vi "Cameras.vi"(4 "error in (no error)":errorcluster, 7 "Image Notifier":refnum<notifier>) -> ()   [LabVIEW 2015]
doc: "This VI runs in parallel to other tasks. It gets images from the camera, processes them for color or shape and use that information to affect robot behavior."
uses:
  <vilib>/Rock Robotics/WPI/Camera/WPI_CameraImageSize.ctl
  Robot Global Data.vi
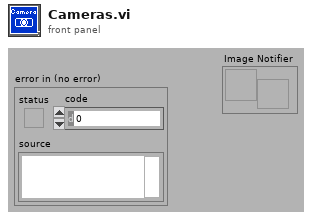
[diagram p1: front panel]
types:
  T1 = typedef "Image Type" = u32
  T2 = typedef "WPI_CameraImageSize.ctl" = enum16{"640x480", "320x240", "160x120", "Custom"}
  T3 = typedef "WPI_CameraDevRef.ctl" = cluster{"Camera Address":string, "CameraStatus":errorcluster}
  T4 = typedef "IMAQ Image.ctl" = refnum<image>
  T5 = enum16{"Update Mode", "Get Image", "Get Image Data"}
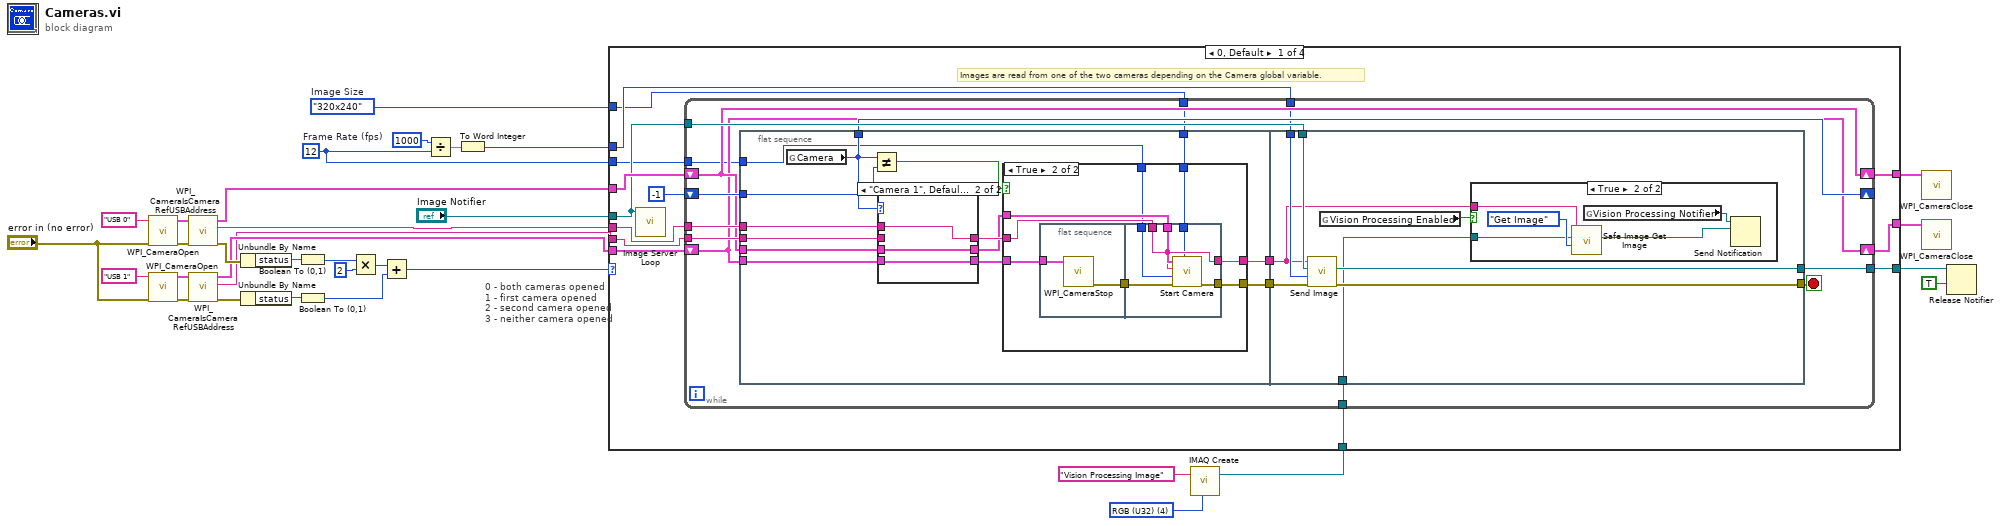
[diagram p0: block diagram]
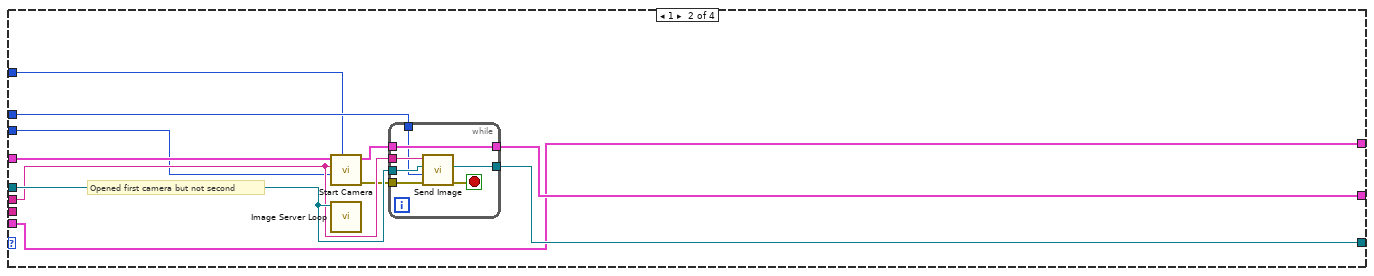
[diagram p5: hidden frame]
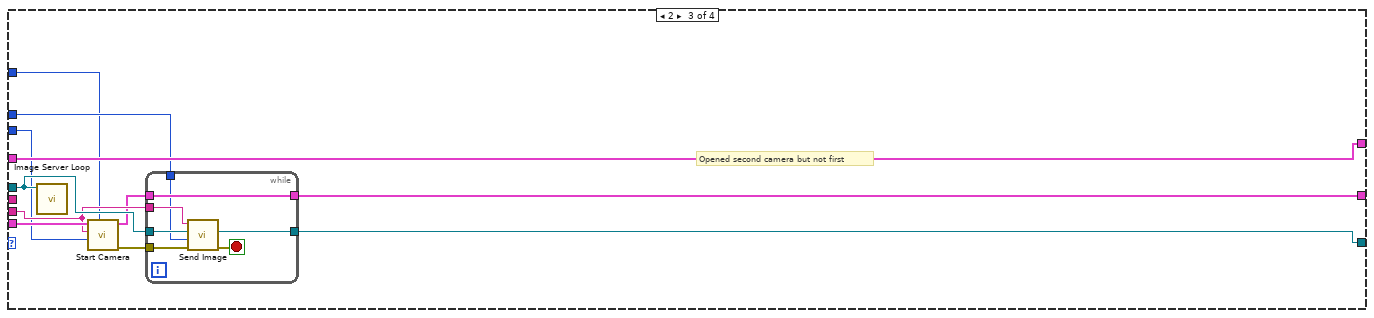
[diagram p6: hidden frame]
diagram:
  w3 = T1 4 items=["Grayscale (U8)", "Grayscale (I16)", "Grayscale (SGL)", "Complex (CSG)", "RGB (U32)", "HSL (U32)", "RGB (U64)", "Grayscale (U16)"] ("Image Type")
  w6 = 12  # Frame Rate (fps)
  w5 = WPI_CameraImageSize."320x240"  # Image Size
  n1 = call <vilib>:"WPI_CameraOpen.vi"("error in (no error)"="error in (no error)", "Camera Address"="USB 0" ("format string")) -> ("error out"=w18:errorcluster, "CameraDevRef"=w20:T3)  [unwired: 8 out]
  n2 = call <vilib>:"WPI_CameraOpen.vi"("error in (no error)"="error in (no error)", "Camera Address"="USB 1" ("format string")) -> ("error out"=w14:errorcluster, "CameraDevRef"=w16:T3)  [unwired: 8 out]
  n3 = call <vilib>:"WPI_CameraIsCameraRefUSBAddress.vi"("error in (no error)"=w18, "CameraDevRef"=w20) -> ("error out"=w17:errorcluster, "Camera Address Out"=w11:string, "CameraDevRef out"=w19:T3)  [unwired: 6 in, 1 out]
  n4 = call <vilib>:"WPI_CameraIsCameraRefUSBAddress.vi"("error in (no error)"=w14, "CameraDevRef"=w16) -> ("error out"=w13:errorcluster, "Camera Address Out"=w12:string, "CameraDevRef out"=w15:T3)  [unwired: 6 in, 1 out]
  n5 = Unbundle By Name(w17) -> ("status"=w9:bool)
  n6 = Unbundle By Name(w13) -> ("status"=w10:bool)
  n7 = Boolean To (0,1)(Boolean=w9) -> (0, 1=w24:i16)
  n8 = Boolean To (0,1)(Boolean=w10) -> (0, 1=w26:i16)
  n9 = Multiply(x=w24, y=i16 2) -> (x*y=w25:i16)
  n10 = Add(x=w25, y=w26) -> (x+y=w28:i16)
  n11 = Divide(x=1000, y=w6) -> (x/y=w7:dbl)
  n12 = To Word Integer(number=w7) -> (16bit integer=w4:i16)
  n13 = call "IMAQ Create"("Image Name"="Vision Processing Image", "Image Type"=w3) -> ("New Image"=w1:T4)  [unwired: 2 in, 2 out]
  n14 = case "0 - both cameras opened\n1 - first camera opened\n2 - second camera opened\n3 - neither camera opened" shown="0, Default" w28 {
    tunnel: [w46 w120 w137 w149] -> w33
    tunnel: "Image Notifier" -> [w39 w121 w139 w148]
    tunnel: [w45 w119 w138 w150] -> w31
    tunnel: w15 -> [w44 w119 w136 w149]
    tunnel: w19 -> [w43 w117 w138 w150]
    tunnel: w12 -> [w42 _ w135 _]
    tunnel: w11 -> [w41 w116 _ _]
    tunnel: [w40 w122 w140 w148] -> w30
    tunnel: w4 -> [w37 w114 w132 _]
    tunnel: w6 -> [w36 w113 w131 _]
    tunnel: w5 -> [w34 w112 w130 _]
    tunnel: w1 -> [w35 _ _ _]
    frame 0, Default {
      # "Images are read from one of the two cameras depending on the Camera global variable."
      n15 = call "Image Server Loop.vi"("Image Notifier"=w39) -> ()  [unwired: 11 in]
      n16 = while {
        shift-right: [w52] -> w46
        shift-left: w44 -> [w52]
        tunnel: w39 -> [w60]
        shift-right: [w53] -> w45
        shift-left: w43 -> [w53]
        tunnel: w42 -> [w56]
        tunnel: w41 -> [w57]
        tunnel: [w61] -> w40
        shift-right: [w55] -> _
        shift-left: -1 -> [w59]
        tunnel: w37 -> [w50]
        tunnel: w36 -> [w49]
        tunnel: w35 -> [w48]
        tunnel: w34 -> [w47]
        stop <- w58 stop-if-true
        n17 = flat-sequence {
          tunnel: w59 -> [w74]
          tunnel: w53 -> [w73]
          tunnel: w52 -> [w72]
          tunnel: w57 -> [w71]
          tunnel: w56 -> [w70]
          tunnel: [w64] -> w55
          tunnel: [w69] -> w54
          tunnel: [w65] -> w51
          tunnel: w49 -> [w63]
          tunnel: w47 -> [w62]
          tunnel: [w106] -> w61
          tunnel: w60 -> [w105]
          tunnel: [w104] -> w58
          tunnel: w54 -> [w103]
          tunnel: w51 -> [w101]
          tunnel: w50 -> [w102]
          tunnel: w48 -> [w100]
          frame #0 {
            n18 = global read "Robot Global Data.vi" "Camera"() -> (w64:enum16{"Camera 1", "Camera 2"})
            n19 = Not Equal?(x=w64, y=w74) -> (x != y?=w75:bool)
            n20 = case shown="\"Camera 1\", Default" w64 {
              tunnel: [w77 w81] -> w66
              tunnel: w72 -> [w78 w81]
              tunnel: [w78 w80] -> w67
              tunnel: w73 -> [w77 w80]
              tunnel: w70 -> [w76 _]
              tunnel: w71 -> [_ w79]
              tunnel: [w76 w79] -> w68
              frame "Camera 2" {
              }
              frame "Camera 1", Default {
              }
            }
            n21 = case shown="True" w75 {
              tunnel: [_ w89] -> w69
              tunnel: w68 -> [w82 w88]
              tunnel: w67 -> [_ w87]
              tunnel: w66 -> [_ w86]
              tunnel: [w82 w85] -> w65
              tunnel: w63 -> [_ w84]
              tunnel: w62 -> [_ w83]
              frame False {
              }
              frame True {
                n22 = flat-sequence {
                  tunnel: [w92] -> w90
                  tunnel: w86 -> [w91]
                  tunnel: w90 -> [w98]
                  tunnel: [w97] -> w89
                  tunnel: w88 -> [w95]
                  tunnel: w87 -> [w96]
                  tunnel: [w95] -> w85
                  tunnel: w84 -> [w94]
                  tunnel: w83 -> [w93]
                  frame #0 {
                    n23 = call <vilib>:"WPI_CameraStop.vi"("CameraDevRef"=w91) -> ("error out"=w92:errorcluster)  [unwired: 9 in, 1 out]
                  }
                  frame #1 {
                    n24 = call "Start Camera.vi"("Image Size"=w93, "error in"=w98, "Frame Rate (fps)"=w94, "Camera Address"=w95, "CameraDevRef"=w96) -> ("error out"=w97:errorcluster)  [unwired: 5 in, 1 out]
                  }
                }
              }
            }
          }
          frame #1 {
            n25 = call "Send Image.vi"("error in (no error)"=w103, "Wait (ms)"=w102, "notifier"=w105, "Camera Address"=w101) -> ("error out"=w104:errorcluster, "notifier out"=w106:refnum<notifier>)  [unwired: 6 in]
            n26 = global read "Robot Global Data.vi" "Vision Processing Enabled"() -> (w99:bool)
            n27 = case shown="True" w99 {
              tunnel: w101 -> [_ w110]
              tunnel: w100 -> [_ w109]
              frame False {
              }
              frame True {
                n28 = call <vilib>:"Safe Image Get Image.vi"("Operation"=T5."Get Image", "Image In"=w109, "Session In"=w110) -> ("Image Out"=w107:T4)  [unwired: 5 in, 3 out]
                n29 = global read "Robot Global Data.vi" "Vision Processing Notifier"() -> (w108:refnum<notifier>)
                n30 = Send Notification(notification=w107, notifier=w108) -> ()  [unwired: 1 in, 2 out]
              }
            }
          }
        }
      }
    }
    frame 1 {
      # "Opened first camera but not second"
      n31 = call "Start Camera.vi"("Image Size"=w112, "Frame Rate (fps)"=w113, "Camera Address"=w116, "CameraDevRef"=w117) -> ("error out"=w115:errorcluster, "CameraDevRef Out"=w118:T3)  [unwired: 6 in]
      n32 = call "Image Server Loop.vi"("Image Notifier"=w121) -> ()  [unwired: 11 in]
      n33 = while {
        tunnel: w121 -> [w129]
        tunnel: w116 -> [w127]
        tunnel: [w128] -> w122
        tunnel: w118 -> [w126]
        tunnel: [w126] -> w120
        tunnel: w115 -> [w124]
        tunnel: w114 -> [w123]
        stop <- w125 stop-if-true
        n34 = call "Send Image.vi"("error in (no error)"=w124, "Wait (ms)"=w123, "notifier"=w129, "Camera Address"=w127) -> ("error out"=w125:errorcluster, "notifier out"=w128:refnum<notifier>)  [unwired: 6 in]
      }
    }
    frame 2 {
      # "Opened second camera but not first"
      n35 = call "Image Server Loop.vi"("Image Notifier"=w139) -> ()  [unwired: 11 in]
      n36 = call "Start Camera.vi"("Image Size"=w130, "Frame Rate (fps)"=w131, "Camera Address"=w135, "CameraDevRef"=w136) -> ("error out"=w133:errorcluster, "CameraDevRef Out"=w134:T3)  [unwired: 6 in]
      n37 = while {
        tunnel: w139 -> [w147]
        tunnel: w135 -> [w145]
        tunnel: [w146] -> w140
        tunnel: w134 -> [w144]
        tunnel: [w144] -> w137
        tunnel: w133 -> [w142]
        tunnel: w132 -> [w141]
        stop <- w143 stop-if-true
        n38 = call "Send Image.vi"("error in (no error)"=w142, "Wait (ms)"=w141, "notifier"=w147, "Camera Address"=w145) -> ("error out"=w143:errorcluster, "notifier out"=w146:refnum<notifier>)  [unwired: 6 in]
      }
    }
    frame 3 {
      # "Failed to open both of the cameras"
    }
  }
  n39 = call <vilib>:"WPI_CameraClose.vi"("CameraDevRef"=w31) -> ()  [unwired: 1 in, 10 out]
  n40 = call <vilib>:"WPI_CameraClose.vi"("CameraDevRef"=w33) -> ()  [unwired: 1 in, 10 out]
  n41 = Release Notifier(notifier=w30, force destroy? (F)=TRUE) -> ()  [unwired: 1 in, 3 out]
